vi "SICK LIDAR.vi"() -> ()   [LabVIEW 2012]
uses:
  <instrlib>/Sick LMS 2XX Series/HAIOL/Sick LMS 2XX Series.lvclass
  <instrlib>/Sick LMS 2XX Series/HAIOL/VISA/Sick LMS 2XX Series VISA.lvclass
panel:
  out "Cartesian Graph":cluster{"X":dbl[], "Y":dbl[]}(graph)
  in  "LMS Type (0: Standard)":u16(ring) items=["Standard", "Non-Standard"]
  out "Polar Co-ordinates":u16[](array[numeric])
  out "Reflectivity Values":i32[](array[numeric])
  in  "Baud Rate":u16(ring) items=["9600", "19200", "38400", "500000"]
  in  "error in":errorcluster
  in  "VISA resource name":refnum<visa-resource-name>
  in  "Debug":bool
  out "error out":errorcluster
  in  "stop?":bool
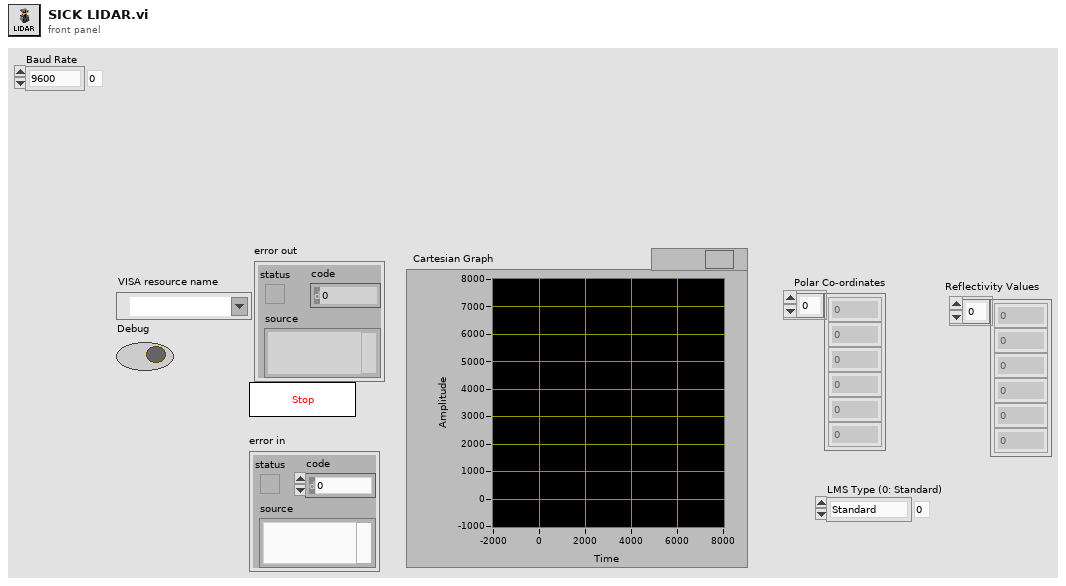
[diagram p1: front panel]
types:
  T1 = cluster{"Reflectivity Values":i32[], "Polar Co-ordinates":u16[]}
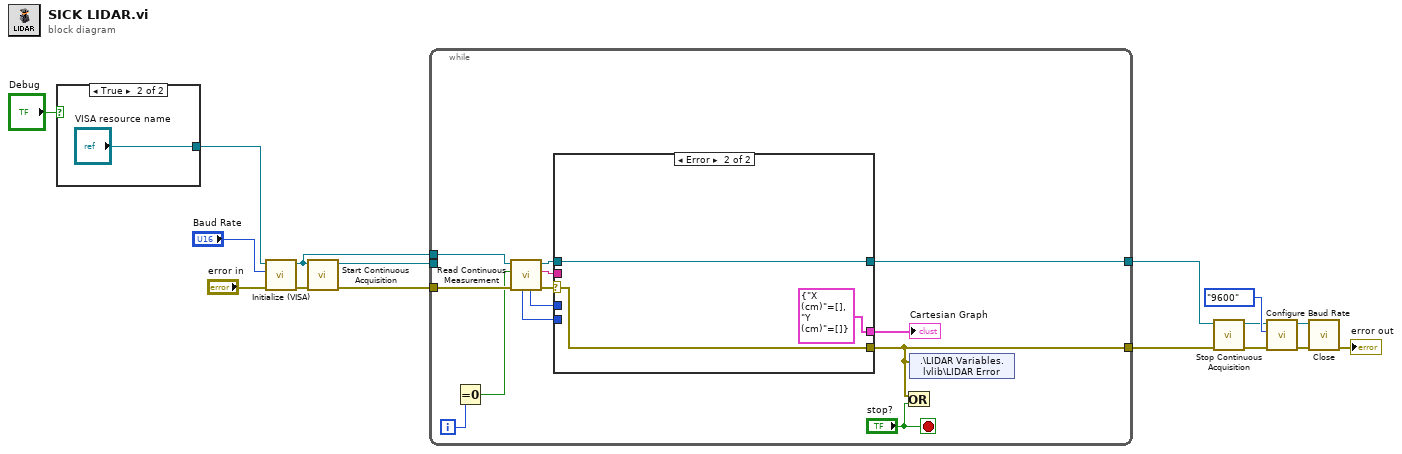
[diagram p0: block diagram]
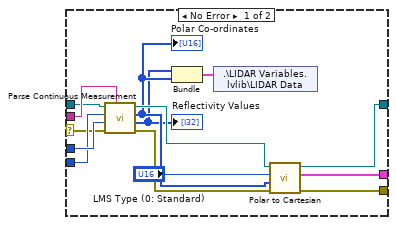
[diagram p2: hidden frame]
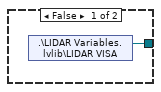
[diagram p3: hidden frame]
diagram:
  n1 = case shown="True" "Debug" {
    tunnel: [w17 "VISA resource name"] -> w12
    frame False {
      n2 = shared-variable ".\\LIDAR Variables.lvlib\\LIDAR VISA"() -> (w17:refnum<visa-resource-name>)  [unwired: 1 in, 1 out]
    }
    frame True {
    }
  }
  n3 = call <instrlib>:"Initialize (VISA).vi"("error in (no error)"="error in", "Baud Rate"="Baud Rate", "VISA resource name"=w12) -> ("error out"=w13:errorcluster, "Sick LMS 2XX Series out"=w1:refnum<class "Sick LMS 2XX Series.lvclass">)  [unwired: 7 in]
  n4 = call-dynamic "Start Continuous Acquisition.vi"("error in (no error)"=w13, "Sick LMS 2XX Series"=w1) -> ("error out"=w15:errorcluster, "Sick LMS 2XX Series out"=w2:refnum<class "Sick LMS 2XX Series.lvclass">)  [unwired: 8 in]
  n5 = while {
    tunnel: [w31] -> w5
    tunnel: w15 -> [w26]
    tunnel: [w28] -> w3
    tunnel: w2 -> [_]
    tunnel: w1 -> [w21]
    i -> [w19]
    stop <- "stop?" stop-if-true
    n6 = Equal To 0?(x=w19) -> (x = 0?=w20:bool)
    n7 = call-dynamic "Read Continuous Measurement.vi"("error in (no error)"=w26, "Enable Acknowledge Byte (T: Enable)"=w20, "Sick LMS 2XX Series"=w21) -> ("error out"=w22:errorcluster, "Read Buffer"=w24:string, "Sick LMS 2XX Series out"=w23:refnum<class "Sick LMS 2XX Series.lvclass">, "Number of Reflectances"=w27:u16, "Number of Distances"=w25:u16)  [unwired: 2 in, 2 out]
    n8 = case shown="Error" w22 {
      selector: w22 -> [w32 w48]
      tunnel: [w36 w48] -> w31
      tunnel: [w43 cluster{"X (cm)":dbl[], "Y (cm)":dbl[]} {"X (cm)"=[], "Y (cm)"=[]} ("Cartesian")] -> w29
      tunnel: [w38 w47] -> w28
      tunnel: w27 -> [w41 _]
      tunnel: w25 -> [w40 _]
      tunnel: w24 -> [w39 _]
      tunnel: w23 -> [w37 w47]
      frame No Error {
        n9 = call-dynamic "Parse Continuous Measurement.vi"("Input Data"=w39, "error in (no error)"=w32, "Number of Reflectances (0)"=w41, "Number of Measurements (1)"=w40, "Sick LMS 2XX Series"=w37) -> ("error out"=w45:errorcluster, "Reflectivity Values"=w33:i32[], "Polar Co-ordinates"=w35:u16[], "Sick LMS 2XX Series out"=w42:refnum<class "Sick LMS 2XX Series.lvclass">)  [unwired: 3 in]
        "Polar Co-ordinates" <- w35
        "Reflectivity Values" <- w33
        n10 = Bundle("Reflectivity Values"=w33, "Polar Co-ordinates"=w35) -> (w34:T1)  [unwired: 1 in]
        n11 = shared-variable ".\\LIDAR Variables.lvlib\\LIDAR Data"(w34) -> ()  [unwired: 1 in, 1 out]
        n12 = call-dynamic "Polar to Cartesian.vi"("error in (no error)"=w45, "Distances"=w35, "LMS Type (0: Standard)"="LMS Type (0: Standard)", "Sick LMS 2XX Series"=w42) -> ("error out"=w36:errorcluster, "Cartesian"=w43:cluster{"X (cm)":dbl[], "Y (cm)":dbl[]}, "Sick LMS 2XX Series out"=w38:refnum<class "Sick LMS 2XX Series.lvclass">)  [unwired: 5 in]
      }
      frame Error {
      }
    }
    "Cartesian Graph" <- w29
    n13 = Or(x=w31, y="stop?") -> ()  [unwired: 1 out]
    n14 = shared-variable ".\\LIDAR Variables.lvlib\\LIDAR Error"(w31) -> ()  [unwired: 1 in, 1 out]
  }
  n15 = call-dynamic "Stop Continuous Acquisition.vi"("error in (no error)"=w5, "Sick LMS 2XX Series"=w3) -> ("error out"=w8:errorcluster, "Sick LMS 2XX Series out"=w9:refnum<class "Sick LMS 2XX Series.lvclass">)  [unwired: 7 in, 1 out]
  n16 = call-dynamic "Configure Baud Rate.vi"("error in (no error)"=w8, "Baud Rate"=enum16{"9600", "19200", "38400", "500000"}."9600" ("Enum"), "Sick LMS 2XX Series"=w9) -> ("error out"=w6:errorcluster, "Sick LMS 2XX Series out"=w7:refnum<class "Sick LMS 2XX Series.lvclass">)  [unwired: 7 in]
  n17 = call-dynamic "Close.vi"("error in (no error)"=w6, "Sick LMS 2XX Series"=w7) -> ("error out"=→"error out":errorcluster)  [unwired: 9 in]
